vi "Get Result.vi"(6 "Last request":bool, 8 "error in (no error)":errorcluster, 11 "Timer in":refnum<class "Timer.lvclass">) -> (0 "error out":errorcluster, 2 "Result":refnum<class "Acquired Result.lvclass">, 3 "Timer out":refnum<class "Timer.lvclass">)   [LabVIEW 2016, in "Timer.lvclass"]
uses:
  Timer.lvclass
  C:/github/LabActor/Worker/Worker.lvclass
  C:/github/LabActor/Template Module/Template Module.lvclass
  NHMFL_Core/Libraries/Instruments/Results/Acquired Result/Acquired Result.lvclass
  Worker/Worker.lvclass/Worker.ctl
  Timer.lvclass/Timer.ctl
  Template Module/Template Module.lvclass/Template Module.ctl
  <vilib>/express/express signal manip/GetorSetDDTAttributes/Shared VIs/TimeType.ctl
  NHMFL_Core/Libraries/Instruments/Results/Acquired Result/Acquired Result.lvclass/Acquired Result.ctl
  Write First call.vi
  NHMFL_Core/Libraries/Instruments/Results/Acquired Result/Write Channels.vi
  NHMFL_Core/Libraries/Instruments/Results/Acquired Result/Write Sender.vi
  NHMFL_Core/Libraries/Instruments/Results/Acquired Result/Write Group.vi
  NHMFL_Core/Libraries/Instruments/Results/Acquired Result/Write Final.vi
  Template Module/Read State.vi
  Read Latest time.vi
  Template Module/Read Name.vi
  Read First call.vi
  Read Start time.vi
  Worker/Read Cycle period.vi
  Write Delay active.vi
  <vilib>/express/express shared/transition.llb/Dynamic To Waveform Array.vi
  <vilib>/express/express signal manip/GetorSetDDTAttributes/Set DDT Attributes/SetT0.vi
  <vilib>/express/express shared/transition.llb/Waveform Array To Dynamic.vi
  <vilib>/express/express signal manip/GetorSetDDTAttributes/Shared VIs/TimeMode Enum to Boolean.vi
  <vilib>/express/express signal manip/GetorSetDDTAttributes/Set DDT Attributes/Set DDT Properties.xnode
  <vilib>/express/express signal manip/GetorSetDDTAttributes/Shared VIs/GetSetShared.lvlib
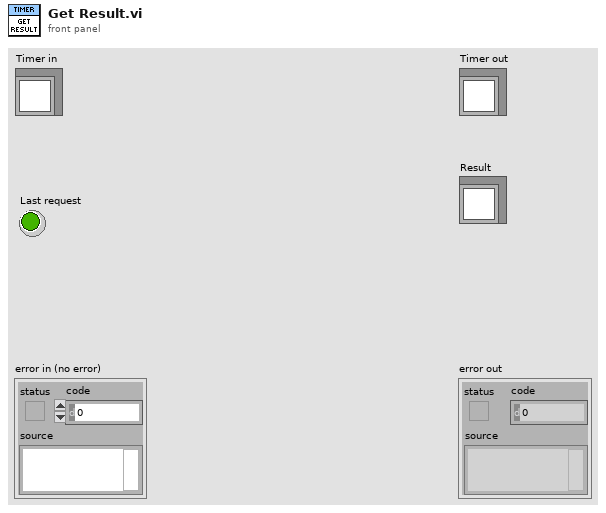
[diagram p1: front panel]
types:
  T1 = typedef "Worker State.ctl" = enum16{"Idle", "Starting", "Working", "Stopping"}
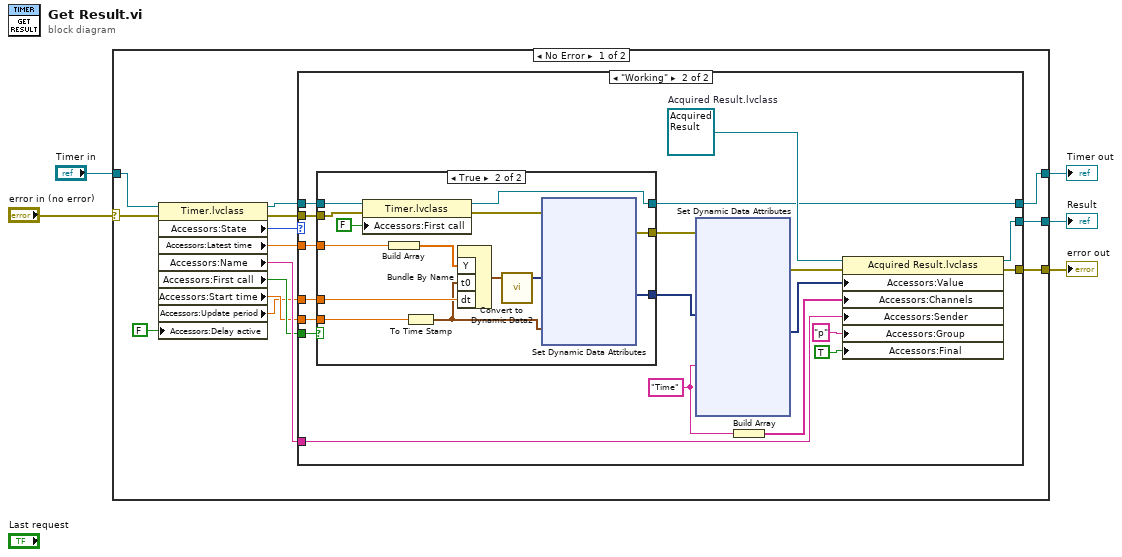
[diagram p0: block diagram]
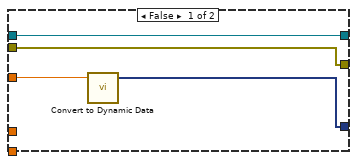
[diagram p3: hidden frame]
diagram:
  n1 = case shown="No Error" "error in (no error)" {
    selector: "error in (no error)" -> [w14 w97]
    tunnel: [w13 w97] -> w1
    tunnel: [w11 w96] -> w2
    tunnel: "Timer in" -> [w19 w96]
    tunnel: [w7 _] -> w3
    frame No Error {
      n2 = property class="Timer.lvclass"(reference=w19, error in=w14, "Accessors:Delay active"=FALSE ("Delay active")) -> (reference out=w12:refnum<class "Timer.lvclass">, error out=w16:errorcluster, "Accessors:State"=w18:T1, "Accessors:Latest time"=w17:dbl, "Accessors:Name"=w15:string, "Accessors:First call"=w10:bool, "Accessors:Start time"=w9:dbl, "Accessors:Update period"=w8:dbl)
      n3 = case shown="\"Working\"" w18 {
        tunnel: w17 -> [_ w38]
        tunnel: w16 -> [w21 w27]
        tunnel: w15 -> [_ w39]
        tunnel: [w21 w23] -> w13
        tunnel: w12 -> [w20 w26]
        tunnel: [w20 w31] -> w11
        tunnel: w10 -> [_ w30]
        tunnel: w9 -> [_ w29]
        tunnel: w8 -> [_ w28]
        tunnel: [_ w22] -> w7
        frame "Idle", Default {
        }
        frame "Working" {
          w35 = "Time" ("String")
          w40 = refnum<class "Acquired Result.lvclass"> refnum  # Acquired Result.lvclass
          n4 = case shown="True" w30 {
            tunnel: w38 -> [w44 w58]
            tunnel: [w43 w48] -> w37
            tunnel: w29 -> [_ w57]
            tunnel: w28 -> [_ w56]
            tunnel: w26 -> [w42 w53]
            tunnel: w27 -> [w41 w52]
            tunnel: [w42 w50] -> w31
            tunnel: [w41 w45] -> w25
            frame False {
              n5 = call "Convert to Dynamic Data"("Double"=w44) -> ("Dynamic Data Type"=w43:dynamicdata)  [unwired: 3 in]
            }
            frame True {
              n6 = property class="Timer.lvclass"(reference=w53, error in=w52, "Accessors:First call"=FALSE ("First call")) -> (reference out=w50:refnum<class "Timer.lvclass">, error out=w46:errorcluster)
              n7 = Build Array(w58) -> (w55:dbl[])
              n8 = To Time Stamp(1:w57) -> (0:w47:timestamp)
              n9 = Bundle By Name("Y"=w55, "t0"=w47, "dt"=w56) -> (w54:waveform(dbl))  [unwired: 1 in]
              n10 = call "Convert to Dynamic Data2"("Waveform"=w54) -> ("Dynamic Data Type"=w49:dynamicdata)  [unwired: 3 in]
              n11 = xnode "Set Dynamic Data Attributes"("Signals In"=w49, "Timestamp"=w47, "error in"=w46) -> ("Signals Out"=w48:dynamicdata, "error out"=w45:errorcluster)  [unwired: 1 in]
            }
          }
          n12 = xnode "Set Dynamic Data Attributes"("Signals In"=w37, "Signal Name"=w35, "error in"=w25) -> ("Signals Out"=w34:dynamicdata, "error out"=w33:errorcluster)  [unwired: 3 in]
          n13 = Build Array(w35) -> (w36:string[])
          n14 = property class="Acquired Result.lvclass"(reference=w40, error in=w33, "Accessors:Value"=w34, "Accessors:Channels"=w36, "Accessors:Sender"=w39, "Accessors:Group"="p" ("Group"), "Accessors:Final"=TRUE ("Final")) -> (reference out=w22:refnum<class "Acquired Result.lvclass">, error out=w23:errorcluster)
        }
      }
    }
    frame Error {
    }
  }
  "error out" <- w1
  "Timer out" <- w2
  "Result" <- w3
